vi "MainT2.vi"() -> ()   [LabVIEW 2019]
uses:
  <instrlib>/niDMM/nidmm.llb/niDMM Function.ctl
  <instrlib>/niDMM/nidmm.llb/niDMM Resolution in Digits.ctl
panel:
  out "time between obtaining data (ms)":u32
  in  "Self-Calibrate Multimeter at the beginning?":bool
  in  "Tab Control":T1(tab)
  out "Waveform Chart 2":cluster{dbl, dbl, dbl}(graph)
  in  "VISA resource name":refnum<visa-resource-name>="COM3"
  in  "termination char\n(0xA = '\\n' = LF)":u8=13 format="%.0x"
  in  "Recieve Data":bool
  out "Thermometer":dbl(slide) scale=0.0..100.0
  in  "physical channels":tag="PXI1Slot2/ai2"
  in  "resistance configuration":i32(ring)=2 items=["2-Wire"=2, "3-Wire"=3, "4-Wire"=4]
  in  "selection":i32
  out "Waveform Chart 4":T2(graph)
  out "Waveform Chart 3":dbl(graph)
  out "Measurement (Volts)":dbl format="%_5p"
  out "Over Range?":bool
  in  "Instrument Descriptor":refnum<k15>="PXI1Slot4"
  in  "Function":T3
  in  "Resolution in Digits":T4=5.5 items=["3 1/2"=3.5, "4 1/2"=4.5, "5 1/2"=5.5, "6 1/2"=6.5, "7 1/2"=7.5]
  in  "Range (Volts)":dbl=10.0 format="%.2p"
  in  "stop program":bool
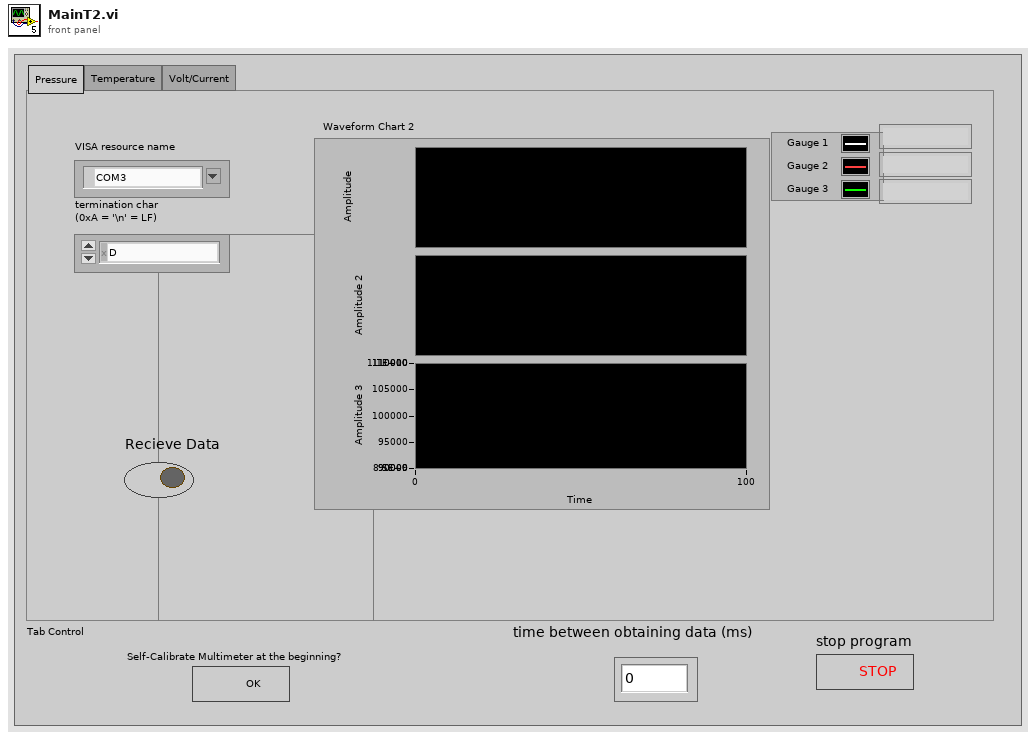
[diagram p1: front panel]
types:
  T1 = enum32{"Pressure", "Temperature", "Volt/Current"}
  T2 = cluster{"data[0]":dbl, "data[1]":dbl, "data[2]":dbl, "data[3]":dbl, "data[4]":dbl, "data[5]":dbl, "data[6]":dbl, "data[7]":dbl, "data[8]":dbl}
  T3 = typedef "niDMM Function.ctl" = enum16{"DC Volts", "AC Volts", "DC Current", "AC Current", "2-wire Resistance", "4-wire Resistance", "Diode", "Frequency", "Period", "AC Volts DC Coupled", "Capacitance", "Inductance", "Temperature"}
  T4 = typedef "niDMM Resolution in Digits.ctl" = dbl
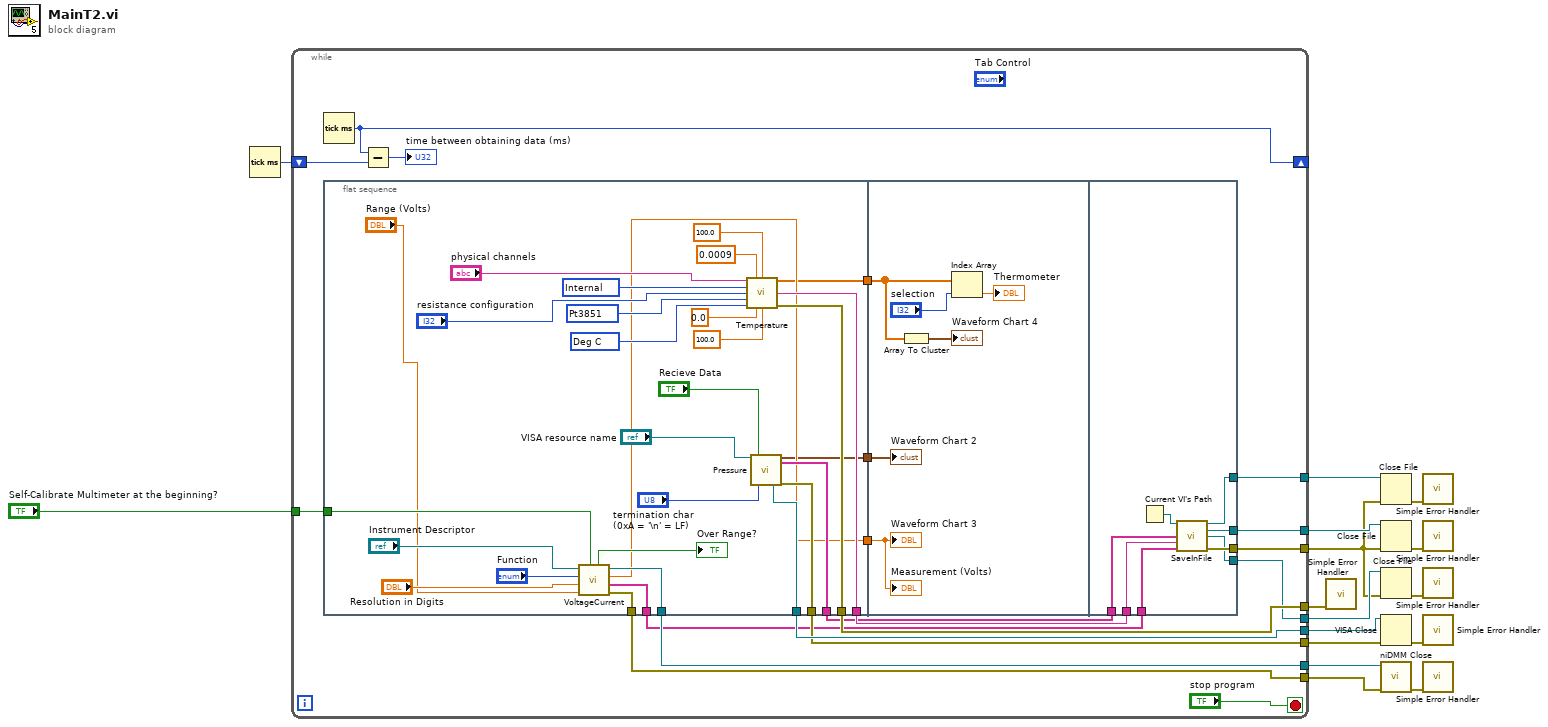
[diagram p0: block diagram]
diagram:
  n1 = Tick Count (ms)() -> (millisecond timer value=w1:u32)
  n2 = while {
    tunnel: [w33] -> w16
    tunnel: [w34] -> w15
    tunnel: [w35] -> w13
    tunnel: "Self-Calibrate Multimeter at the beginning?" -> [w32]
    tunnel: [w30] -> w10
    tunnel: [w31] -> w9
    tunnel: [w25] -> w2
    tunnel: [w24] -> w5
    tunnel: [w23] -> w4
    tunnel: [w22] -> w3
    shift-right: [w19] -> _
    shift-left: w1 -> [w18]
    stop <- "stop program" stop-if-true
    n3 = Tick Count (ms)() -> (millisecond timer value=w19:u32)
    n4 = flat-sequence {
      tunnel: [w56] -> w28
      tunnel: [w55] -> w35
      tunnel: [w52] -> w34
      tunnel: [w51] -> w27
      tunnel: [w50] -> w33
      tunnel: w32 -> [w46]
      tunnel: [w45] -> w31
      tunnel: [w44] -> w30
      tunnel: [w43] -> w29
      tunnel: [w41] -> w26
      tunnel: [w39] -> w21
      tunnel: [w38] -> w20
      tunnel: w29 -> [w70]
      tunnel: w21 -> [w69]
      tunnel: w20 -> [w67]
      tunnel: w28 -> [w77]
      tunnel: w27 -> [w78]
      tunnel: w26 -> [w76]
      tunnel: [w75] -> w25
      tunnel: [w74] -> w24
      tunnel: [w73] -> w23
      tunnel: [w72] -> w22
      frame #0 {
        w59 = 10143 items=["Deg C"=10143, "Deg F"=10144, "Kelvins"=10325, "Deg R"=10145, "From Custom Scale"=10065] ("units")
        w60 = 10071 items=["Pt3750"=12481, "Pt3851"=10071, "Pt3911"=12482, "Pt3916"=10069, "Pt3920"=10053, "Pt3928"=12483, "Custom"=10137] ("rtd type")
        w61 = 10200 items=["Internal"=10200, "External"=10167, "None"=10230] ("current excitation source")
        n5 = call "VoltageCurrent.vi"("Self-Calibrate at the beginning?"=w46, "Range (Volts)"="Range (Volts)", "Resolution in Digits"="Resolution in Digits", "Function"="Function", "Instrument Descriptor"="Instrument Descriptor") -> ("error out"=w45:errorcluster, "output array"=w41:string[], "Measurement (Volts)"=w43:dbl, "instrument handle out"=w44:refnum<k15>, "Over Range?"=→"Over Range?":bool)  [unwired: 2 in]
        n6 = call "Temperature.vi"("physical channels"="physical channels", "current excitation value"=0.0009, "r0"=100.0, "current excitation source"=w61, "resistance configuration"="resistance configuration", "rtd type"=w60, "units"=w59, "minimum value"=0.0, "maximum value"=100.0) -> ("data"=w39:dbl[], "spreadsheet string"=w56:string, "error out"=w55:errorcluster)  [unwired: 4 in]
        n7 = call "Pressure.vi"("VISA resource name"="VISA resource name", "Recieve Data"="Recieve Data", "termination char\n(0xA = '\\n' = LF)"="termination char\n(0xA = '\\n' = LF)") -> ("VISA resource name out"=w52:refnum<visa-resource-name>, "output cluster"=w38:cluster{dbl, dbl, dbl}, "output array"=w51:string[], "error out"=w50:errorcluster)  [unwired: 10 in, 3 out]
      }
      frame #1 {
        n8 = Array To Cluster(array=w69) -> (cluster=→"Waveform Chart 4":T2)
        n9 = Index Array(array=w69, index="selection") -> (element=→"Thermometer":dbl)
        "Waveform Chart 3" <- w70
        "Measurement (Volts)" <- w70
        "Waveform Chart 2" <- w67
      }
      frame #2 {
        n10 = Current VI's Path() -> (path=w79:path)
        n11 = call "SaveInFile.vi"("path"=w79, "pressureData"=w78, "tempData"=w77, "4071data"=w76) -> ("refnum out"=w74:refnum<file>, "refnum out 2"=w73:refnum<file>, "refnum out 3"=w72:refnum<file>, "error out"=w75:errorcluster)  [unwired: 8 in]
      }
    }
    n12 = Subtract(x=w19, y=w18) -> (x-y=→"time between obtaining data (ms)":u32)
  }
  n13 = call <vilib>:"Simple Error Handler.vi"("error in (no error)"=w13) -> ()  [unwired: 4 in, 5 out]
  n14 = Close File(refnum=w5, error in=w2) -> (error out=w6:errorcluster)  [unwired: 1 out]
  n15 = Close File(refnum=w4, error in=w2) -> (error out=w7:errorcluster)  [unwired: 1 out]
  n16 = Close File(refnum=w3, error in=w2) -> (error out=w12:errorcluster)  [unwired: 1 out]
  n17 = VISA Close(VISA resource name=w15, error in (no error)=w16) -> (error out=w14:errorcluster)
  n18 = call <instrlib>:"niDMM Close.vi"("error in (no error)"=w9, "instrument handle"=w10) -> ("error out"=w8:errorcluster)  [unwired: 9 in]
  n19 = call <vilib>:"Simple Error Handler.vi"("error in (no error)"=w6) -> ()  [unwired: 1 in, 8 out]
  n20 = call <vilib>:"Simple Error Handler.vi"("error in (no error)"=w7) -> ()  [unwired: 1 in, 8 out]
  n21 = call <vilib>:"Simple Error Handler.vi"("error in (no error)"=w12) -> ()  [unwired: 1 in, 8 out]
  n22 = call <vilib>:"Simple Error Handler.vi"("error in (no error)"=w14) -> ()  [unwired: 4 in, 5 out]
  n23 = call <vilib>:"Simple Error Handler.vi"("error in (no error)"=w8) -> ()  [unwired: 4 in, 5 out]
